vi "SetAcceleration.vi"(8 "error in":errorcluster, 9 "Acceleration":dbl, 10 "Axial #":i32, 11 "VISA resource":refnum<visa-resource-name>) -> (0 "error out":errorcluster)   [LabVIEW 2012, in "ESP300.lvlib"]
uses:
  <instrlib>/ESP300/ESP300.lvlib
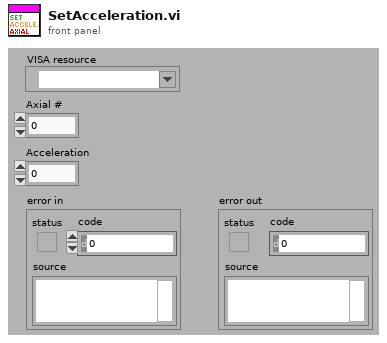
[diagram p1: front panel]
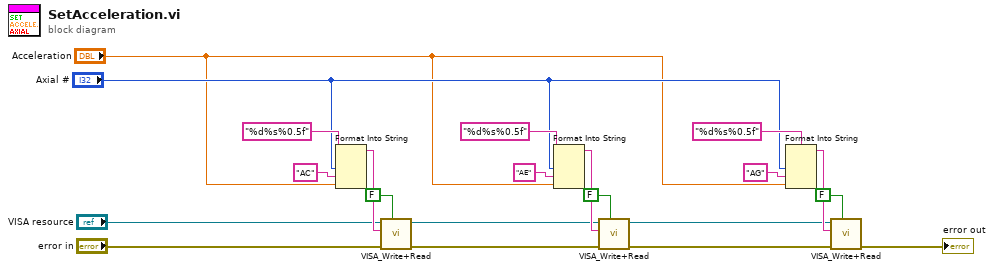
[diagram p0: block diagram]
diagram:
  n1 = Format Into String(format string="%d%s%0.5f", "Axial #", "AC" ("input 2"), "Acceleration") -> (resulting string=w16:string)  [unwired: 2 in, 1 out]
  n2 = call <instrlib>:"VISA_Write+Read.vi"("Read?"=FALSE, "error in (no error)"="error in", "Write Buffer"=w16, "VISA resource name"="VISA resource") -> ("error out"=w9:errorcluster)  [unwired: 5 in, 2 out]
  n3 = Format Into String(format string="%d%s%0.5f", "Axial #", "AE" ("input 2"), "Acceleration") -> (resulting string=w15:string)  [unwired: 2 in, 1 out]
  n4 = call <instrlib>:"VISA_Write+Read.vi"("Read?"=FALSE, "error in (no error)"=w9, "Write Buffer"=w15, "VISA resource name"="VISA resource") -> ("error out"=w8:errorcluster)  [unwired: 5 in, 2 out]
  n5 = Format Into String(format string="%d%s%0.5f", "Axial #", "AG" ("input 2"), "Acceleration") -> (resulting string=w10:string)  [unwired: 2 in, 1 out]
  n6 = call <instrlib>:"VISA_Write+Read.vi"("Read?"=FALSE, "error in (no error)"=w8, "Write Buffer"=w10, "VISA resource name"="VISA resource") -> ("error out"=→"error out":errorcluster)  [unwired: 5 in, 2 out]
